vi "Reset.vi"(8 "error in":errorcluster, 11 "Configuration UI in":refnum<class "Configuration UI.lvclass">) -> (0 "error out":errorcluster, 3 "Configuration UI out":refnum<class "Configuration UI.lvclass">)   [LabVIEW 2023, in "Configuration UI.lvlib" / "Configuration UI.lvclass"]
doc: "Call <b>Select Instrument</b> index 0"
uses:
  Project/Configuration UI.lvclass
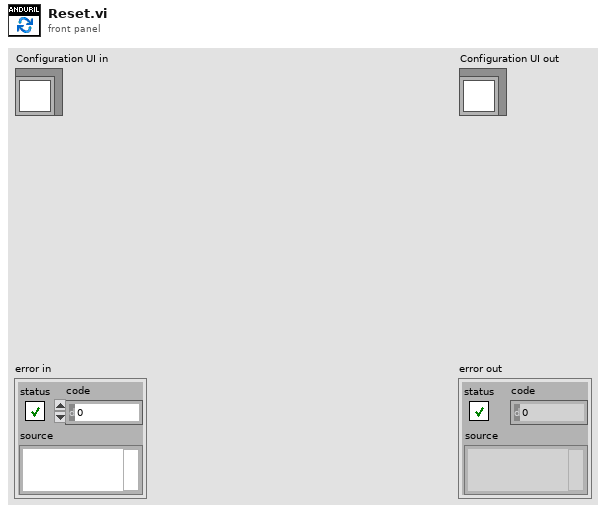
[diagram p1: front panel]
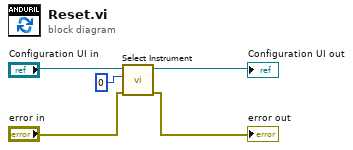
[diagram p0: block diagram]
diagram:
  n1 = call "Select Instrument.vi"("error in (no error)"="error in", "Selected"=0, "Configuration UI in"="Configuration UI in") -> ("error out"=→"error out":errorcluster, "Configuration UI out"=→"Configuration UI out":refnum<class "Configuration UI.lvclass">)  [unwired: 7 in]
